vi "Interpolate 2D Scattered_Evaluate.vi"(6 "Length":dbl[](array[numeric]), 8 "area":dbl, 9 "W":dbl[](array[numeric]), 10 "Y":dbl[](array[numeric]), 11 "X":dbl[](array[numeric])) -> (0 "M":dbl[](array[numeric]), 1 "N3":dbl[](array[numeric]), 2 "N2":dbl[](array[numeric]), 3 "N1":dbl[](array[numeric]))   [LabVIEW 2017, in "NI_AAL_Interpolation.lvlib"]
uses:
  <vilib>/gmath/NI_AAL_Interpolation.lvlib
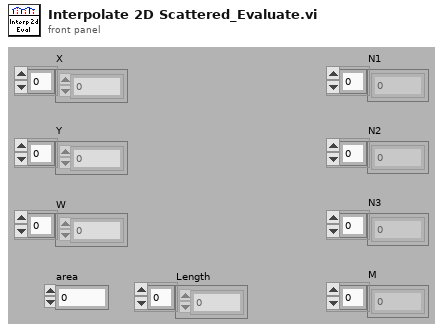
[diagram p1: front panel]
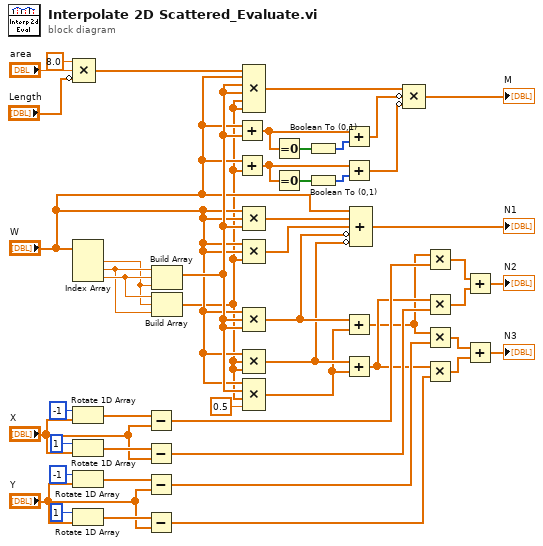
[diagram p0: block diagram]
diagram:
  n1 = Compound Arithmetic op=MULTIPLY(8.0, "area", invert "Length") -> (w17:dbl[])
  n2 = Index Array(array="W") -> (element #1=w47:dbl, element #2=w48:dbl, element #3=w49:dbl)  [unwired: 3 in]
  n3 = Rotate 1D Array(1:"X", 2:-1 ("n")) -> (0:w43:dbl[])
  n4 = Rotate 1D Array(1:"X", 2:1 ("n")) -> (0:w44:dbl[])
  n5 = Rotate 1D Array(1:"Y", 2:-1 ("n")) -> (0:w41:dbl[])
  n6 = Rotate 1D Array(1:"Y", 2:1 ("n")) -> (0:w40:dbl[])
  n7 = Subtract(x=w43, y="X") -> (x-y=w31:dbl[])
  n8 = Subtract(x=w44, y="X") -> (x-y=w30:dbl[])
  n9 = Subtract(x=w41, y="Y") -> (x-y=w27:dbl[])
  n10 = Subtract(x=w40, y="Y") -> (x-y=w26:dbl[])
  n11 = Build Array(w48, w49, w47) -> (w16:dbl[])
  n12 = Build Array(w49, w47, w48) -> (w13:dbl[])
  n13 = Add(x="W", y=w16) -> (x+y=w7:dbl[])
  n14 = Add(x="W", y=w13) -> (x+y=w10:dbl[])
  n15 = Compound Arithmetic op=MULTIPLY(w17, "W", w16, w16, w13, w13) -> (w6:dbl[])
  n16 = Compound Arithmetic op=MULTIPLY("W", "W", w16) -> (w15:dbl[])
  n17 = Compound Arithmetic op=MULTIPLY("W", "W", w13) -> (w36:dbl[])
  n18 = Compound Arithmetic op=MULTIPLY("W", w16, w16) -> (w34:dbl[])
  n19 = Compound Arithmetic op=MULTIPLY("W", w13, w13) -> (w33:dbl[])
  n20 = Compound Arithmetic op=MULTIPLY("W", w16, w13, 0.5) -> (w32:dbl[])
  n21 = Equal To 0?(x=w7) -> (x = 0?=w8:bool[])
  n22 = Equal To 0?(x=w10) -> (x = 0?=w12:bool[])
  n23 = Boolean To (0,1)(Boolean=w8) -> (0, 1=w9:i16[])
  n24 = Boolean To (0,1)(Boolean=w12) -> (0, 1=w11:i16[])
  n25 = Add(x=w7, y=w9) -> (x+y=w5:dbl[])
  n26 = Add(x=w10, y=w11) -> (x+y=w4:dbl[])
  n27 = Add(x=w34, y=w32) -> (x+y=w1:dbl[])
  n28 = Add(x=w33, y=w32) -> (x+y=w2:dbl[])
  n29 = Compound Arithmetic op=ADD("W", w15, w36, invert w34, invert w33) -> (→"N1":dbl[])
  n30 = Compound Arithmetic op=MULTIPLY(w6, invert w5, invert w4) -> (→"M":dbl[])
  n31 = Multiply(x=w1, y=w31) -> (x*y=w28:dbl[])
  n32 = Multiply(x=w2, y=w30) -> (x*y=w29:dbl[])
  n33 = Multiply(x=w1, y=w27) -> (x*y=w25:dbl[])
  n34 = Multiply(x=w2, y=w26) -> (x*y=w24:dbl[])
  n35 = Add(x=w28, y=w29) -> (x+y=→"N2":dbl[])
  n36 = Add(x=w25, y=w24) -> (x+y=→"N3":dbl[])
